vi "cm2nm_Delete_sample_location_from_array.vi"(5 "Sample Set In":T1, 6 "Index2Delete":u32, 7 "Sample locations of Interest":refnum<vi>) -> (0 "Sample Set Out":T1, 2 "XY_graphOut":cluster{dbl[], dbl[]}[](array[cluster]))   [LabVIEW 2011]
uses:
  cm2nm_sample_set.ctl
  cm2nm_coordinate_information_v2.ctl
  Instrument_type_enum_v2.ctl
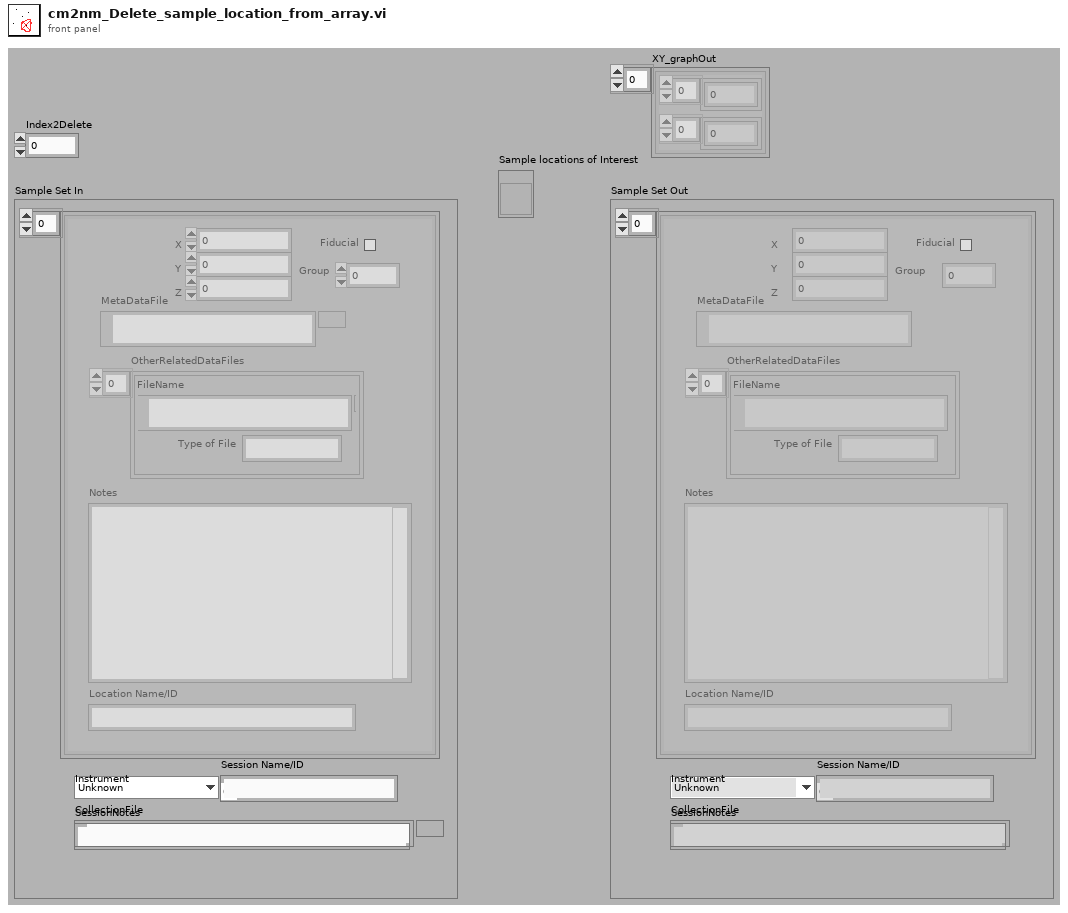
[diagram p1: front panel]
types:
  T1 = typedef "cm2nm_sample_set.ctl" = cluster{"CollectionOfPoints":T2[], "Instrument":T3, "CollectionFile":path, "Session Name/ID":string, "SessionNotes":string}
  T2 = typedef "cm2nm_coordinate_information_v2.ctl" = cluster{"MetaDataFile":path, "X":dbl, "Y":dbl, "Z":dbl, "Group":i32, "Rotation":dbl[unit], "Fiducial":bool, "Magnification":dbl, "Working_Distance":dbl, "Notes":string, "Location Name/ID":string, "OtherRelatedDataFiles":cluster{"Type of File":string, "FileName":path}[], "Available":bool}
  T3 = typedef "Instrument_type_enum_v2.ctl" = enum16{"Unknown", "Philips FEI SEM IRC", "JEOL 7000F EML_MFC", "MXRD MFC", "JEOL_EPMA"}
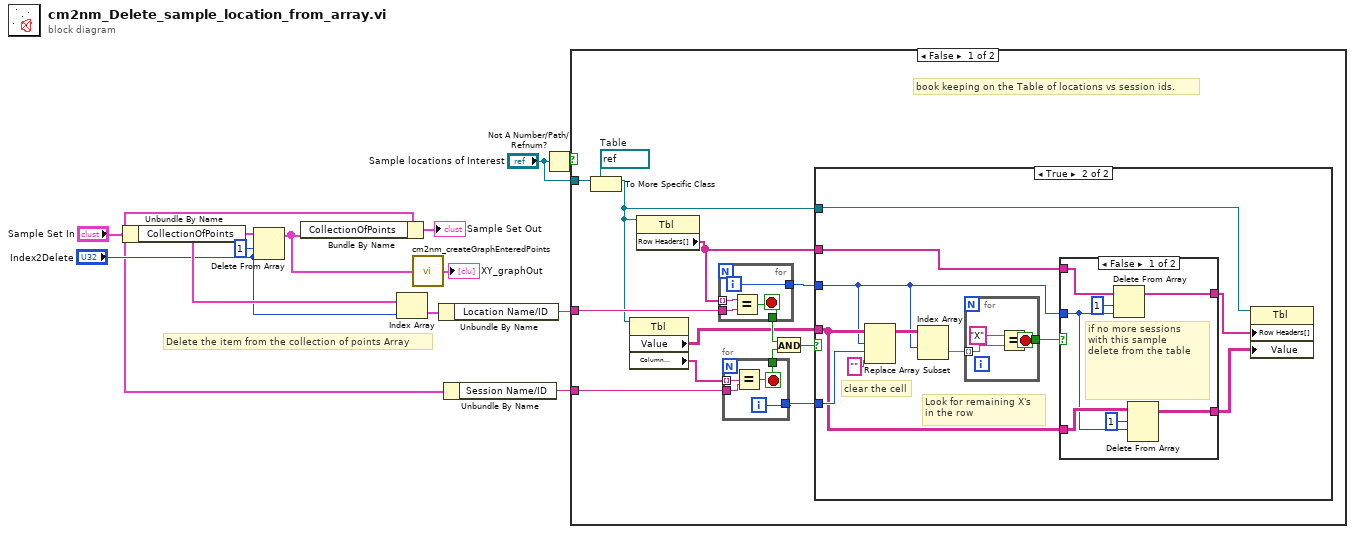
[diagram p0: block diagram]
diagram:
  # "Delete the item from the collection of points Array"
  n1 = Unbundle By Name("Sample Set In") -> ("CollectionOfPoints"=w8:T2[])
  n2 = Delete From Array(array=w8, length=1, index="Index2Delete") -> (array with subset deleted=w12:T2[])  [unwired: 1 out]
  n3 = Bundle By Name(cluster="Sample Set In", "CollectionOfPoints"=w12) -> (→"Sample Set Out":T1)
  n4 = Index Array(array=w8, index="Index2Delete") -> (element=w6:T2)
  n5 = call "cm2nm_createGraphEnteredPoints.vi"("EnteredPoints_in"=w12) -> ("XY_graphOut"=→"XY_graphOut":cluster{dbl[], dbl[]}[])
  n6 = Unbundle By Name(w6) -> ("Location Name/ID"=w3:string)
  n7 = Unbundle By Name("Sample Set In") -> ("Session Name/ID"=w4:string)
  n8 = Not A Number/Path/Refnum?(number/path/refnum="Sample locations of Interest") -> (NaN/Path/Refnum?=w2:bool)
  n9 = case shown="False" w2 {
    tunnel: "Sample locations of Interest" -> [w16 _]
    tunnel: w4 -> [w23 _]
    tunnel: w3 -> [w24 _]
    frame False {
      w13 = refnum<vi> refnum  # Table
      # "book keeping on the Table of locations vs session ids."
      n10 = To More Specific Class(target class=w13, reference=w16) -> (specific class reference=w15:refnum<vi>)  [unwired: 1 in, 1 out]
      n11 = property class="Tbl"(reference=w15) -> ("Value"=w17:string[][], "Column Headers[]"=w25:string[])  [unwired: 1 in, 2 out]
      n12 = property class="Tbl"(reference=w15) -> ("Row Headers[]"=w14:string[])  [unwired: 1 in, 2 out]
      n13 = for {
        tunnel: w24 -> [w56]
        tunnel: w14 -> [w55] mode=indexing
        tunnel: [w54] -> w22
        tunnel: [w53] -> w18
        i -> [w53]
        stop <- w54 stop-if-true
        n14 = Equal?(x=w55, y=w56) -> (x = y?=w54:bool)
      }
      n15 = for {
        tunnel: w25 -> [w52] mode=indexing
        tunnel: w23 -> [w51]
        tunnel: [w50] -> w21
        tunnel: [w49] -> w19
        i -> [w49]
        stop <- w50 stop-if-true
        n16 = Equal?(x=w52, y=w51) -> (x = y?=w50:bool)
      }
      n17 = And(x=w22, y=w21) -> (x .and. y?=w20:bool)
      n18 = case shown="True" w20 {
        tunnel: w19 -> [_ w36]
        tunnel: w18 -> [_ w29]
        tunnel: w17 -> [_ w30]
        tunnel: w14 -> [_ w31]
        tunnel: w15 -> [_ w27]
        frame False {
          # "If can't find the row and the collumn then the x doesn't exist\nshould probably toss a warning to the user here."
        }
        frame True {
          # "Look for remaining X's\nin the row"
          # "clear the cell"
          n19 = Replace Array Subset(array=w30, new element="" ("new element/subarray"), index (row)=w29, index (col)=w36) -> (w34:string[][])
          n20 = Index Array(array=w34, index (row)=w29) -> (element=w33:string[])  [unwired: 1 in]
          n21 = for {
            tunnel: w33 -> [w48] mode=indexing
            tunnel: [w46] -> w32
            stop <- w46 stop-if-true
            n22 = Equal?(x="X", y=w48) -> (x = y?=w46:bool)
          }
          n23 = case shown="False" w32 {
            tunnel: w31 -> [w43 w45]
            tunnel: w30 -> [w40 w44]
            tunnel: w29 -> [w39 _]
            tunnel: [w41 w45] -> w28
            tunnel: [w38 w44] -> w26
            frame False {
              # "if no more sessions\nwith this sample\ndelete from the table"
              n24 = Delete From Array(array=w43, length=1, index=w39) -> (array with subset deleted=w41:string[])  [unwired: 1 out]
              n25 = Delete From Array(array=w40, length=1, index (row)=w39) -> (array with subset deleted=w38:string[][])  [unwired: 1 in, 1 out]
            }
            frame True {
            }
          }
          n26 = property class="Tbl"(reference=w27, "Row Headers[]"=w28, "Value"=w26) -> ()  [unwired: 1 in, 2 out]
        }
      }
    }
    frame True {
      # "This vi can be used from routines that do not have the table\nif the reference is not valid don't do anything."
    }
  }
